vi "Clusters.vi"() -> ()   [LabVIEW 2020]
panel:
  out "Output bbn":T1
  out "output from bundle":T1
  out "Numeric 2":dbl
  out "String":string
  out "Boolean":bool
  out "Numeric":dbl
  in  "Cluster":T1
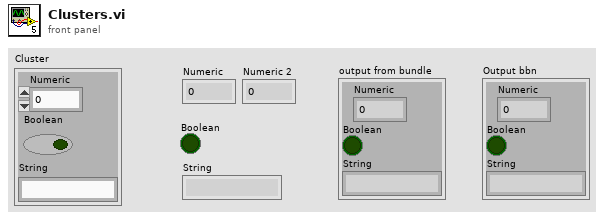
[diagram p1: front panel]
types:
  T1 = cluster{"Numeric":dbl, "Boolean":bool, "String":string}
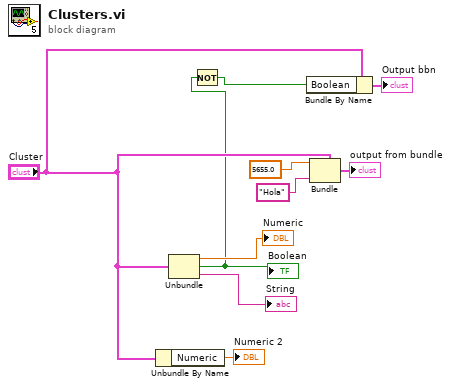
[diagram p0: block diagram]
diagram:
  n1 = Unbundle By Name("Cluster") -> ("Numeric"=→"Numeric 2":dbl)
  n2 = Unbundle("Cluster") -> ("Numeric"=→"Numeric":dbl, "Boolean"=w3:bool, "String"=→"String":string)
  "Boolean" <- w3
  n3 = Not(x=w3) -> (.not. x?=w2:bool)
  n4 = Bundle By Name(cluster="Cluster", "Boolean"=w2) -> (→"Output bbn":T1)
  n5 = Bundle(cluster="Cluster", "Numeric"=5655.0, "String"="Hola") -> (→"output from bundle":T1)  [unwired: 1 in]
